vi "GetSRBody.vi"(8 "Error In":errorcluster, 11 "SR #":string) -> (0 "Error Out":errorcluster, 1 "SR Notes":string[](array[string]), 2 "Documents Used":string[][](array[string]), 3 "Documents Marked as Solution":string[][](array[string]))   [LabVIEW 2017, in "DS_Lib.lvlib" / "SRNotesParser.lvlib"]
uses:
  SRNotesParser.lvlib
  <vilib>/httpClient/LabVIEWHTTPClient.lvlib
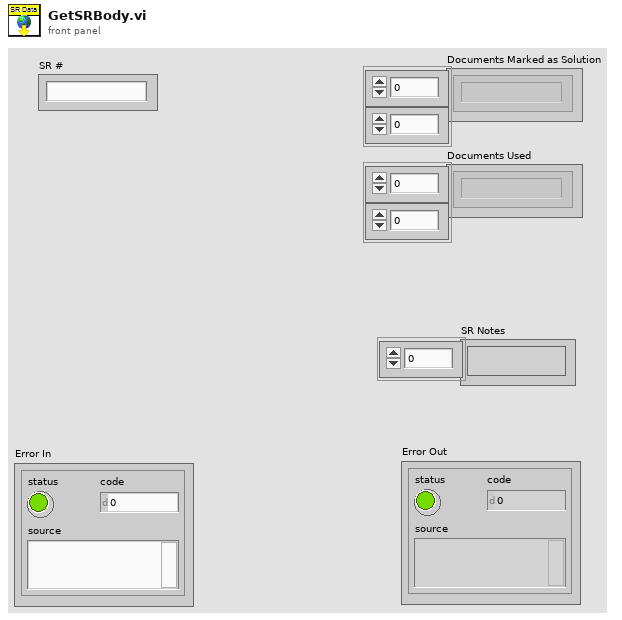
[diagram p1: front panel]
types:
  T1 = typedef "LabVIEWHTTPClient.lvlib/ClientHandle.ctl" = refnum<k1>
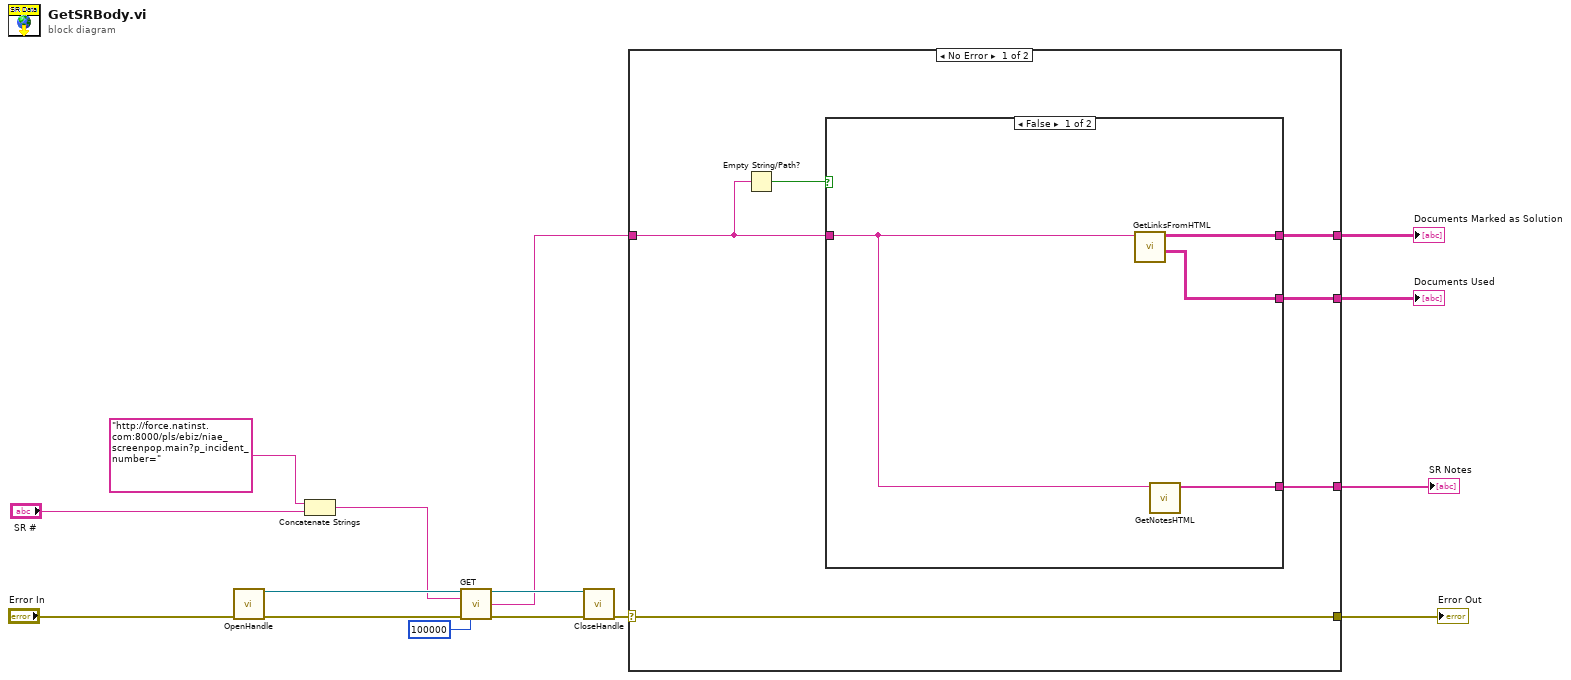
[diagram p0: block diagram]
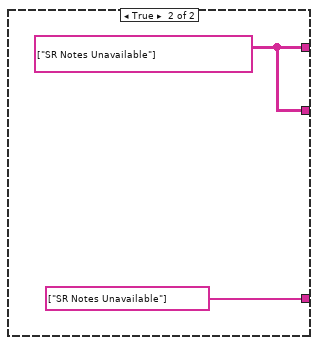
[diagram p2: hidden frame]
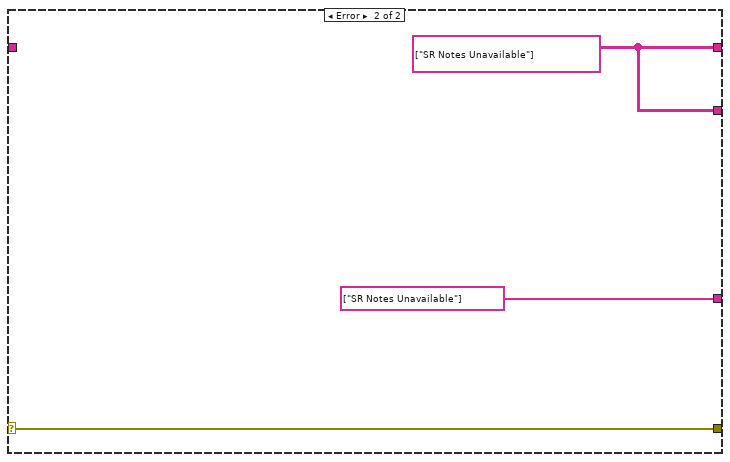
[diagram p3: hidden frame]
diagram:
  n1 = call <vilib>:"OpenHandle.vi"("error in (no error)"="Error In") -> ("client handle out"=w13:T1, "error out"=w12:errorcluster)  [unwired: 13 in]
  n2 = Concatenate Strings("http://force.natinst.com:8000/pls/ebiz/niae_screenpop.main?p_incident_number=" ("command line"), "SR #") -> (w8:string)
  n3 = call <vilib>:"GET.vi"("client handle"=w13, "url"=w8, "error in (no error)"=w12, "timeout (10000)"=100000) -> ("client handle out"=w10:T1, "body"=w6:string, "error out"=w11:errorcluster)  [unwired: 8 in, 1 out]
  n4 = call <vilib>:"CloseHandle.vi"("client handle"=w10, "error in (no error)"=w11) -> ("error out"=w4:errorcluster)  [unwired: 13 in]
  n5 = case shown="No Error" w4 {
    selector: w4 -> [w20 w29]
    tunnel: [w21 string[] ["SR Notes Unavailable"] ("Array")] -> w15
    tunnel: w6 -> [w18 _]
    tunnel: [w20 w29] -> w14
    tunnel: [w17 w28] -> w2
    tunnel: [w16 w28] -> w1
    frame No Error {
      n6 = Empty String/Path?(string/path=w18) -> (empty?=w19:bool)
      n7 = case shown="False" w19 {
        tunnel: [w24 string[] ["SR Notes Unavailable"] ("Array")] -> w21
        tunnel: w18 -> [w25 _]
        tunnel: [w23 w26] -> w17
        tunnel: [w22 w26] -> w16
        frame False {
          n8 = call "GetLinksFromHTML.vi"("SR XML in"=w25) -> ("Documents Used"=w22:string[][], "Documents Marked as Solution"=w23:string[][])  [unwired: 7 in, 2 out]
          n9 = call "GetNotesHTML.vi"("text"=w25) -> ("Array"=w24:string[])  [unwired: 10 in]
        }
        frame True {
          w26 = string[][] [["SR Notes Unavailable"]] ("Solutions Linked")
        }
      }
    }
    frame Error {
      w28 = string[][] [["SR Notes Unavailable"]] ("Solutions Linked")
    }
  }
  "SR Notes" <- w15
  "Error Out" <- w14
  "Documents Marked as Solution" <- w2
  "Documents Used" <- w1
